vi "RowColor.vi"(8 "Customer":string, 9 "Row":i32, 10 "tested":dbl=1.0, 11 "Input":dbl) -> (1 "FontColor":u32, 2 "bgcolor":u32, 3 "ActiveCell":T1)   [LabVIEW 2012]
uses:
  <vilib>/Utility/miscctls.llb/LVRowAndColumnTypeDef.ctl
panel:
  in  "Active Cell:Active Cell":T1
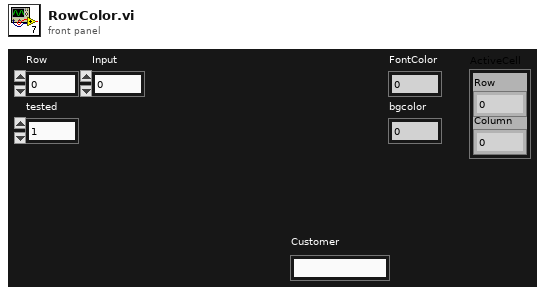
[diagram p1: front panel]
types:
  T1 = typedef "LVRowAndColumnTypeDef.ctl" = cluster{"Row":i32, "Column":i32}
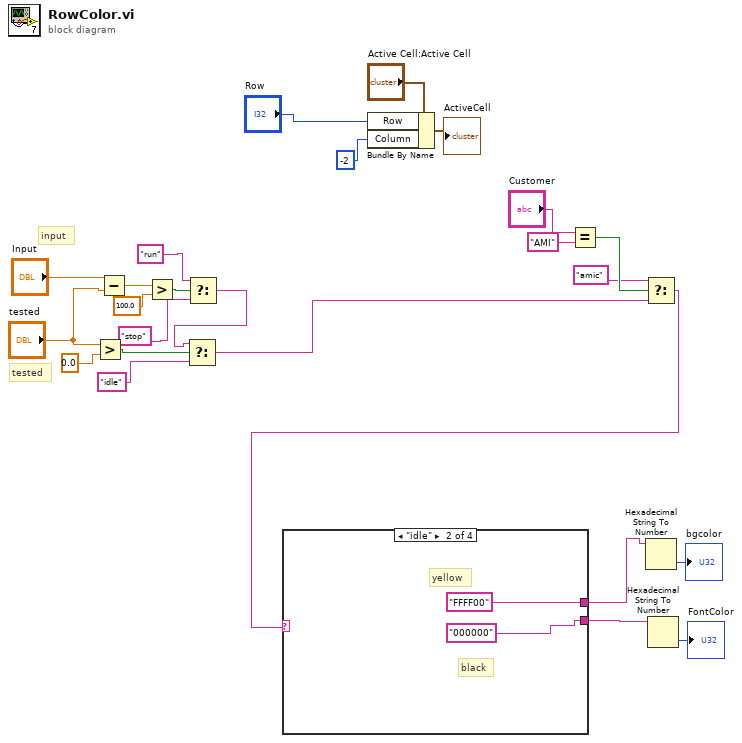
[diagram p0: block diagram]
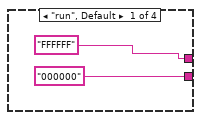
[diagram p2: hidden frame]
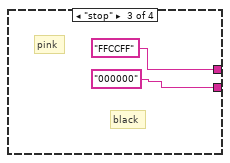
[diagram p3: hidden frame]
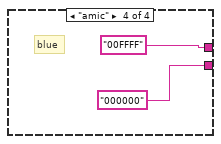
[diagram p4: hidden frame]
diagram:
  # "tested"
  # "input"
  n1 = Greater?(x="tested", y=0.0) -> (0:w15:bool)
  n2 = Subtract(x="Input", y="tested") -> (x-y=w12:dbl)
  n3 = Greater?(x=w12, y=100.0) -> (0:w9:bool)
  n4 = Select(t="run", s=w9, f="stop" ("t")) -> (s? t:f=w1:string)
  n5 = Select(t=w1, s=w15, f="idle") -> (s? t:f=w2:string)
  n6 = Bundle By Name(cluster="Active Cell:Active Cell", "Row"="Row", "Column"=-2 ("element")) -> (→"ActiveCell":T1)
  n7 = Equal?(x="Customer", y="AMI") -> (x = y?=w17:bool)
  n8 = Select(t="amic", s=w17, f=w2) -> (s? t:f=w4:string)
  n9 = case shown="\"idle\"" w4 {
    tunnel: ["000000" "000000" "000000" "000000"] -> w7
    tunnel: ["FFFFFF" "FFFF00" "FFCCFF" "00FFFF" ("y")] -> w6
    frame "run", Default {
    }
    frame "idle" {
      # "black"
      # "yellow"
    }
    frame "stop" {
      # "pink"
      # "black"
    }
    frame "amic" {
      # "blue"
    }
  }
  n10 = Hexadecimal String To Number(string=w6) -> (number=→"bgcolor":u32)  [unwired: 2 in, 1 out]
  n11 = Hexadecimal String To Number(string=w7) -> (number=→"FontColor":u32)  [unwired: 2 in, 1 out]
